vi "SQM160 Comm.vi"() -> (0 "TEMPSTRG":string="!#@O7")   [LabVIEW 2023]
panel:
  out "Shutter":bool
  out "COMPLETE MESSAGE 9":string
  out "CRC2 6":string
  out "CRC1 6":string
  out "Boolean array 6":bool[](array[boolean])
  in  "CRC 14":i16 format="%.0x"
  in  "TEMPCRC 6":i16=16383 format="%.0x"
  out "x-y*floor(x/y) 6":i32
  out "floor(x/y) 6":i32
  out "TEMPSTRG 9":string="!#@O7"
  out "COMPLETE MESSAGE 6":string
  out "CRC2 5":string
  out "CRC1 5":string
  out "Boolean array 5":bool[](array[boolean])
  in  "CRC 11":i16 format="%.0x"
  in  "TEMPCRC 5":i16=16383 format="%.0x"
  out "x-y*floor(x/y) 5":i32
  out "floor(x/y) 5":i32
  out "TEMPSTRG 7":string="!#@O7"
  out "CRC2 4":string
  out "CRC1 4":string
  out "Boolean array 4":bool[](array[boolean])
  in  "CRC 8":i16 format="%.0x"
  in  "TEMPCRC 4":i16=16383 format="%.0x"
  out "x-y*floor(x/y) 4":i32
  out "floor(x/y) 4":i32
  out "TEMPSTRG 5":string="!#@O7"
  out "error code 8":i32 format="%.0x"
  out "error code 7":i32
  out "COMPLETE MESSAGE 4":string
  out "COMPLETE MESSAGE 3":string
  out "CRC2 3":string
  out "CRC1 3":string
  out "Boolean array 3":bool[](array[boolean])
  in  "CRC 5":i16 format="%.0x"
  in  "TEMPCRC 3":i16=16383 format="%.0x"
  out "x-y*floor(x/y) 3":i32
  out "floor(x/y) 3":i32
  out "TEMPSTRG 3":string="!#@O7"
  out "error code 6":i32 format="%.0x"
  out "error code 5":i32
  out "COMPLETE MESSAGE 2":string
  out "CRC2 2":string
  out "CRC1 2":string
  out "TEMPSTRG 2":string="!#@O7"
  out "Boolean array 2":bool[](array[boolean])
  out "first subarray 2":bool[](array[boolean])
  out "second subarray 2":bool[](array[boolean])
  in  "CRC 2":i16 format="%.0x"
  in  "TEMPCRC 2":i16=16383 format="%.0x"
  out "x-y*floor(x/y) 2":i32
  out "floor(x/y) 2":i32
  in  "CH2 FREQUENCY CMD":string="P2"
  in  "CH1 FREQUENCY CMD":string="P1"
  in  "CH2 THICNESS CMD":string="N2"
  in  "CH1 THICKNESS CMD":string="N1"
  in  "CH2  RATE CMD":string="L2"
  out "STATUS":string
  out "error code 4":i32
  out "THICKNESS 2":string="N/A"
  out "FREQUENCY 2":string="N/A"
  out "RATE 2":string="N/A"
  out "FREQUENCY 1":string="N/A"
  out "THICNESS 1":string="N/A"
  out "RATE 1":string="N/A"
  in  "START/STOP":bool
  in  "BAUD RATE":u16(ring)=3 items=["2400", "4800", "9600", "19200", "38400"]
  out "Output Array":string[](array[string])
  out "error code 3":i32 format="%.0x"
  out "error code 2":i32
  out "error code":i32
  in  "COM PORT":u16(ring) items=["COM 1", "COM 2"]
  in  "INIT PORT":bool
  out "COMPLETE MESSAGE":string
  out "CRC2":string
  out "floor(x/y)":i32
  out "x-y*floor(x/y)":i32
  out "CRC1":string
  out "second subarray":bool[](array[boolean])
  out "first subarray":bool[](array[boolean])
  out "Boolean array":bool[](array[boolean])
  in  "CH1 RATE CMD":string="L1"
  in  "TEMPCRC":i16=16383 format="%.0x"
  in  "CRC":i16 format="%.0x"
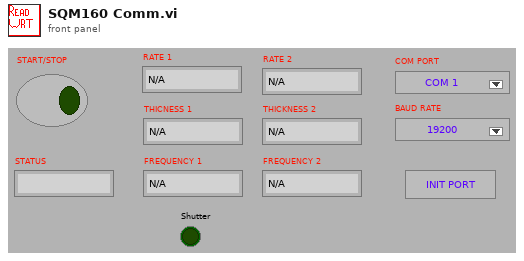
[diagram p1: front panel]
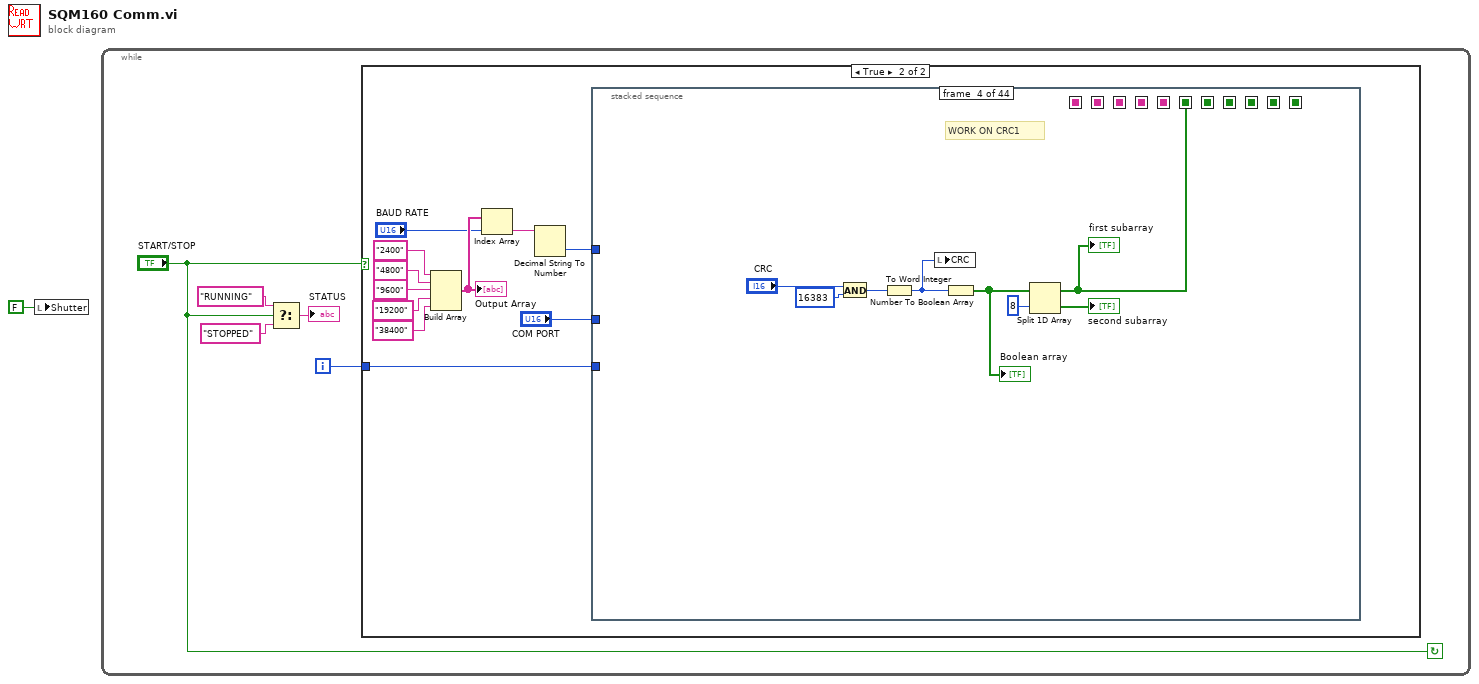
[diagram p0: block diagram]
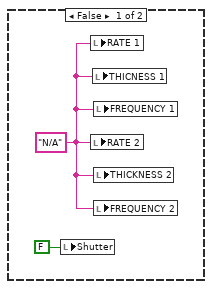
[diagram p2: hidden frame]
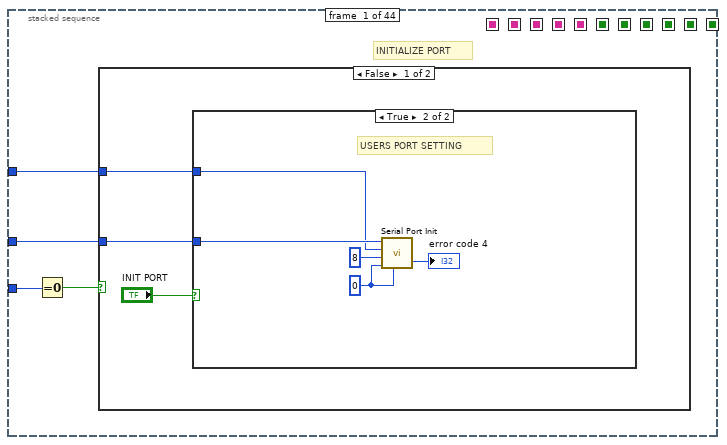
[diagram p3: hidden frame]
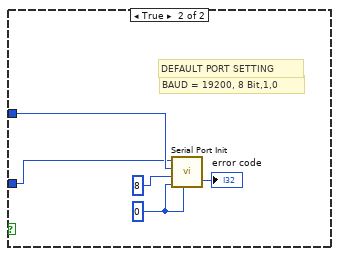
[diagram p5: hidden frame]
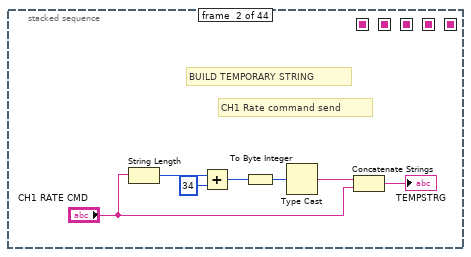
[diagram p6: hidden frame]
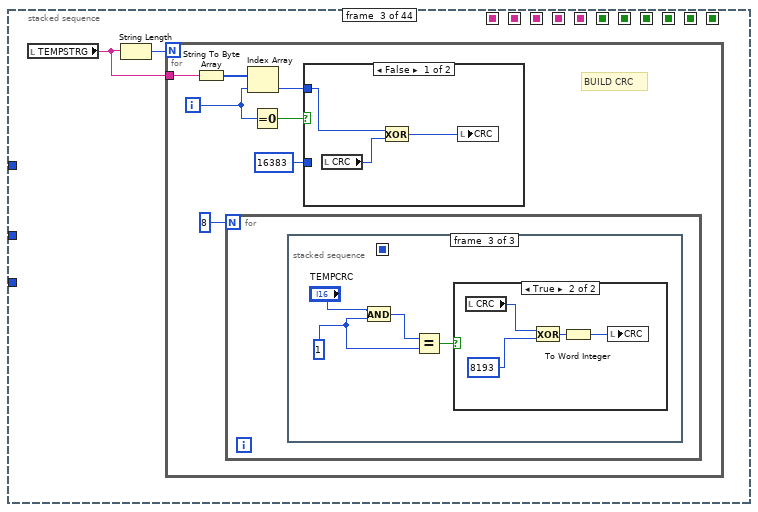
[diagram p7: hidden frame]
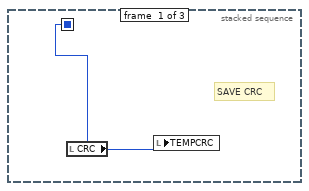
[diagram p8: hidden frame]
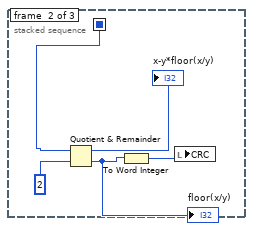
[diagram p9: hidden frame]
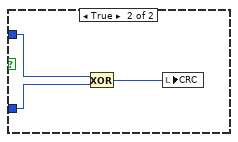
[diagram p11: hidden frame]
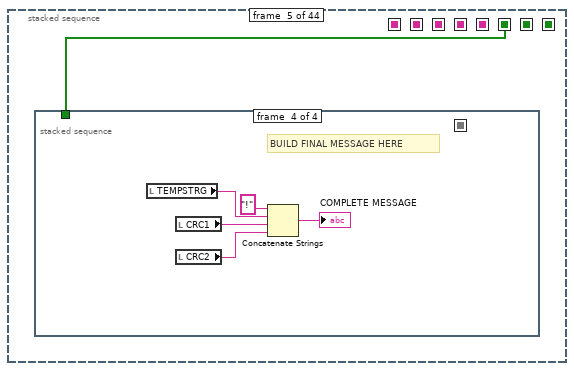
[diagram p12: hidden frame]
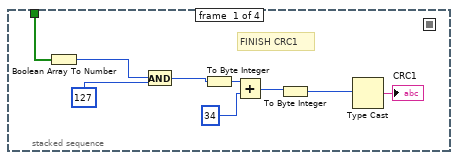
[diagram p13: hidden frame]
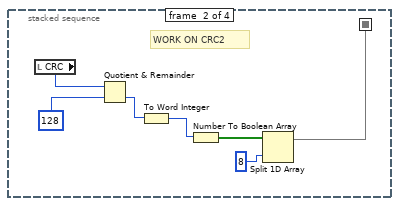
[diagram p14: hidden frame]
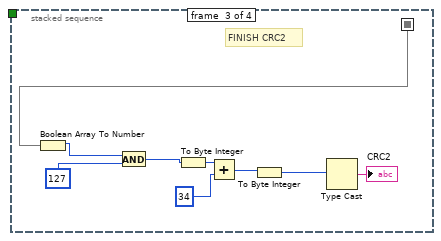
[diagram p15: hidden frame]
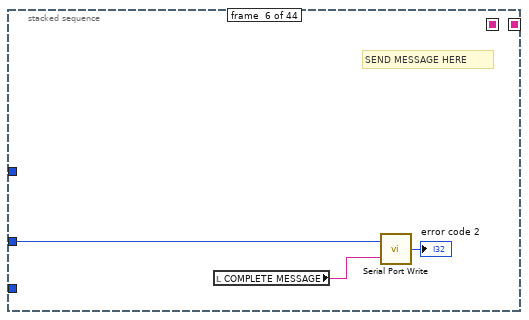
[diagram p16: hidden frame]
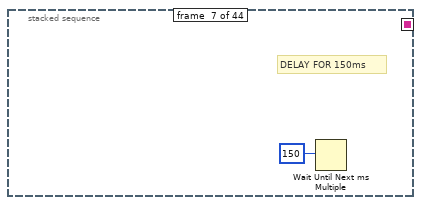
[diagram p17: hidden frame]
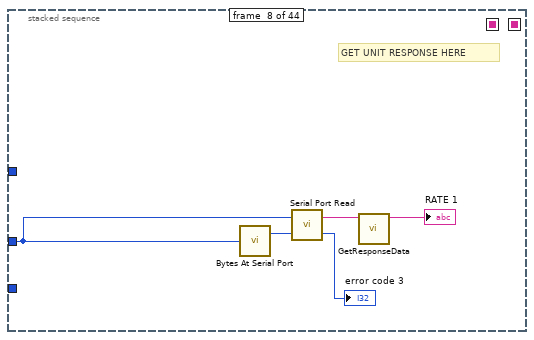
[diagram p18: hidden frame]
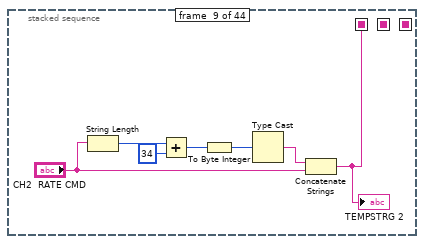
[diagram p19: hidden frame]
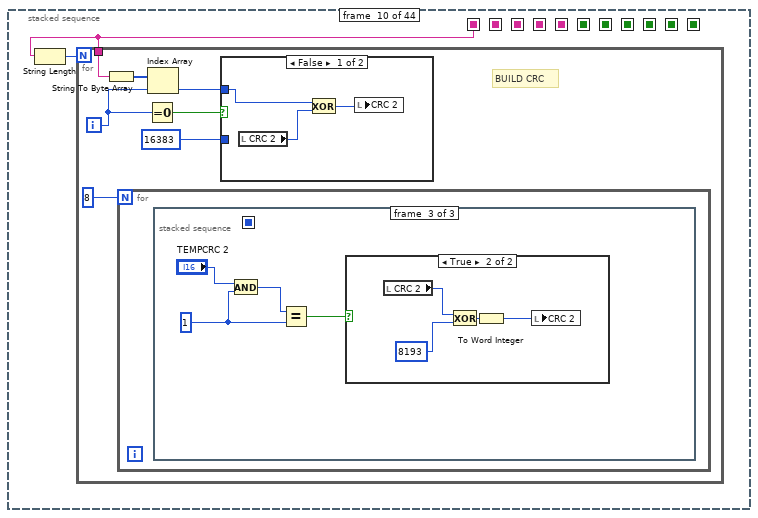
[diagram p20: hidden frame]
diagram:
  n1 = local write "Shutter"(FALSE ("Shutter")) -> ()
  n2 = while {
    i -> [w6]
    stop <- "START/STOP" continue-if-true
    n3 = Select(t="RUNNING", s="START/STOP", f="STOPPED") -> (s? t:f=→"STATUS":string)
    n4 = case shown="True" "START/STOP" {
      tunnel: w6 -> [_ w18]
      frame False {
        w8 = "N/A"
        n5 = local write "Shutter"(FALSE ("Shutter")) -> ()
        n6 = local write "RATE 1"(w8) -> ()
        n7 = local write "RATE 2"(w8) -> ()
        n8 = local write "THICNESS 1"(w8) -> ()
        n9 = local write "FREQUENCY 1"(w8) -> ()
        n10 = local write "THICKNESS 2"(w8) -> ()
        n11 = local write "FREQUENCY 2"(w8) -> ()
      }
      frame True {
        n12 = Build Array("2400", "4800", "9600", "19200", "38400") -> (w12:string[])
        "Output Array" <- w12
        n13 = Index Array(array=w12, index="BAUD RATE") -> (element=w11:string)
        n14 = Decimal String To Number(string=w11) -> (number=w9:i32)  [unwired: 2 in, 1 out]
        n15 = stacked-sequence {
          seq-local: [_ _ _ w77 _ _ _ _ _ _ _ _ _ _ _ _ _ _ _ _ _ _ _ _ _ _ _ _ _ _ _ _ _ _ _ _ _ _ _ _ _ _ _ _] -> [_ _ _ _ w81 _ _ _ _ _ _ _ _ _ _ _ _ _ _ _ _ _ _ _ _ _ _ _ _ _ _ _ _ _ _ _ _ _ _ _ _ _ _ _]
          seq-local: [_ _ _ _ _ _ _ _ w121 _ _ _ _ _ _ _ _ _ _ _ _ _ _ _ _ _ _ _ _ _ _ _ _ _ _ _ _ _ _ _ _ _ _ _] -> [_ _ _ _ _ _ _ _ _ w128 _ _ _ _ _ _ _ _ _ _ _ _ _ _ _ _ _ _ _ _ _ _ _ _ _ _ _ _ _ _ _ _ _ _]
          seq-local: [_ _ _ _ _ _ _ _ _ _ w159 _ _ _ _ _ _ _ _ _ _ _ _ _ _ _ _ _ _ _ _ _ _ _ _ _ _ _ _ _ _ _ _ _] -> [_ _ _ _ _ _ _ _ _ _ _ w165 _ _ _ _ _ _ _ _ _ _ _ _ _ _ _ _ _ _ _ _ _ _ _ _ _ _ _ _ _ _ _ _]
          seq-local: [_ _ _ _ _ _ _ _ _ _ _ _ _ _ _ w206 _ _ _ _ _ _ _ _ _ _ _ _ _ _ _ _ _ _ _ _ _ _ _ _ _ _ _ _] -> [_ _ _ _ _ _ _ _ _ _ _ _ _ _ _ _ w212 _ _ _ _ _ _ _ _ _ _ _ _ _ _ _ _ _ _ _ _ _ _ _ _ _ _ _]
          seq-local: [_ _ _ _ _ _ _ _ _ _ _ _ _ _ _ _ _ w242 _ _ _ _ _ _ _ _ _ _ _ _ _ _ _ _ _ _ _ _ _ _ _ _ _ _] -> [_ _ _ _ _ _ _ _ _ _ _ _ _ _ _ _ _ _ w248 _ _ _ _ _ _ _ _ _ _ _ _ _ _ _ _ _ _ _ _ _ _ _ _ _]
          seq-local: [_ _ _ _ _ _ _ _ _ _ _ _ _ _ _ _ _ _ _ _ _ _ w288 _ _ _ _ _ _ _ _ _ _ _ _ _ _ _ _ _ _ _ _ _] -> [_ _ _ _ _ _ _ _ _ _ _ _ _ _ _ _ _ _ _ _ _ _ _ w295 _ _ _ _ _ _ _ _ _ _ _ _ _ _ _ _ _ _ _ _]
          seq-local: [_ _ _ _ _ _ _ _ _ _ _ _ _ _ _ _ _ _ _ _ _ _ _ _ w325 _ _ _ _ _ _ _ _ _ _ _ _ _ _ _ _ _ _ _] -> [_ _ _ _ _ _ _ _ _ _ _ _ _ _ _ _ _ _ _ _ _ _ _ _ _ w331 _ _ _ _ _ _ _ _ _ _ _ _ _ _ _ _ _ _]
          seq-local: [_ _ _ _ _ _ _ _ _ _ _ _ _ _ _ _ _ _ _ _ _ _ _ _ _ _ _ _ _ w369 _ _ _ _ _ _ _ _ _ _ _ _ _ _] -> [_ _ _ _ _ _ _ _ _ _ _ _ _ _ _ _ _ _ _ _ _ _ _ _ _ _ _ _ _ _ w376 _ _ _ _ _ _ _ _ _ _ _ _ _]
          seq-local: [_ _ _ _ _ _ _ _ _ _ _ _ _ _ _ _ _ _ _ _ _ _ _ _ _ _ _ _ _ _ _ w406 _ _ _ _ _ _ _ _ _ _ _ _] -> [_ _ _ _ _ _ _ _ _ _ _ _ _ _ _ _ _ _ _ _ _ _ _ _ _ _ _ _ _ _ _ _ w412 _ _ _ _ _ _ _ _ _ _ _]
          seq-local: [_ _ _ _ _ _ _ _ _ _ _ _ _ _ _ _ _ _ _ _ _ _ _ _ _ _ _ _ _ _ _ _ _ _ _ _ w450 _ _ _ _ _ _ _] -> [_ _ _ _ _ _ _ _ _ _ _ _ _ _ _ _ _ _ _ _ _ _ _ _ _ _ _ _ _ _ _ _ _ _ _ _ _ w457 _ _ _ _ _ _]
          seq-local: [_ _ _ _ _ _ _ _ _ _ _ _ _ _ _ _ _ _ _ _ _ _ _ _ _ _ _ _ _ _ _ _ _ _ _ _ _ _ w488 _ _ _ _ _] -> [_ _ _ _ _ _ _ _ _ _ _ _ _ _ _ _ _ _ _ _ _ _ _ _ _ _ _ _ _ _ _ _ _ _ _ _ _ _ _ w493 _ _ _ _]
          tunnel: "COM PORT" -> [w23 _ _ _ _ w112 _ w118 _ _ _ _ w196 _ w202 _ _ _ _ w279 _ w285 _ _ _ _ w362 _ w368 _ _ _ _ w443 _ w448 _ _ _ _ w524 _ w529 w531]
          tunnel: w18 -> [w22 _ _ _ _ _ _ _ _ _ _ _ _ _ _ _ _ _ _ _ _ _ _ _ _ _ _ _ _ _ _ _ _ _ _ _ _ _ _ _ _ _ _ _]
          tunnel: w9 -> [w20 _ _ _ _ _ _ _ _ _ _ _ _ _ _ _ _ _ _ _ _ _ _ _ _ _ _ _ _ _ _ _ _ _ _ _ _ _ _ _ _ _ _ _]
          frame #0 {
            # "INITIALIZE PORT"
            n16 = Equal To 0?(x=w22) -> (x = 0?=w21:bool)
            n17 = case shown="False" w21 {
              tunnel: w20 -> [w24 w36]
              tunnel: w23 -> [w25 w34]
              frame False {
                n18 = case shown="True" "INIT PORT" {
                  tunnel: w25 -> [_ w28]
                  tunnel: w24 -> [_ w27]
                  frame False {
                  }
                  frame True {
                    w30 = 0
                    # "USERS PORT SETTING"
                    n19 = call <vilib>:"Serial Port Init.vi"("parity"=w30, "stop bits"=w30, "data bits"=8, "baud rate"=w27, "port number"=w28) -> ("error code"=→"error code 4":i32)  [unwired: 2 in]
                  }
                }
              }
              frame True {
                w33 = 0
                # "BAUD = 19200, 8 Bit,1,0"
                # "DEFAULT PORT SETTING"
                n20 = call <vilib>:"Serial Port Init.vi"("parity"=w33, "stop bits"=w33, "data bits"=8, "baud rate"=w36, "port number"=w34) -> ("error code"=→"error code":i32)  [unwired: 2 in]
              }
            }
          }
          frame #1 {
            # "CH1 Rate command send"
            # "BUILD TEMPORARY STRING"
            n21 = String Length(string="CH1 RATE CMD") -> (length=w43:i32)
            n22 = Add(x=w43, y=34) -> (x+y=w39:i32)
            n23 = To Byte Integer(number=w39) -> (8bit integer=w40:i8)
            n24 = Type Cast(x=w40) -> (*(type *) &x=w38:string)  [unwired: 1 in]
            n25 = Concatenate Strings(w38, "CH1 RATE CMD") -> (→"TEMPSTRG":string)
          }
          frame #2 {
            n26 = local read "TEMPSTRG"() -> (w45:string)
            n27 = String Length(string=w45) -> (length=w44:i32)
            n28 = for {
              N: w44 -> [_]
              tunnel: w45 -> [w49]
              i -> [w52]
              # "BUILD CRC"
              n29 = String To Byte Array(string=w49) -> (unsigned byte array=w48:u8[])
              n30 = for {
                N: 8 -> [_]
                n31 = stacked-sequence {
                  seq-local: [w53 _ _] -> [_ w58 _]
                  frame #0 {
                    # "SAVE CRC"
                    n32 = local read "CRC"() -> (w53:i16)
                    n33 = local write "TEMPCRC"(w53) -> ()
                  }
                  frame #1 {
                    n34 = Quotient & Remainder(x=w58, y=2) -> (x-y*floor(x/y)=→"x-y*floor(x/y)":i32, floor(x/y)=w54:i32)
                    "floor(x/y)" <- w54
                    n35 = To Word Integer(number=w54) -> (16bit integer=w56:i16)
                    n36 = local write "CRC"(w56) -> ()
                  }
                  frame #2 {
                    w60 = 1
                    n37 = And(x="TEMPCRC", y=w60) -> (x .and. y?=w61:i32)
                    n38 = Equal?(x=w61, y=w60) -> (x = y?=w59:bool)
                    n39 = case shown="True" w59 {
                      frame False {
                      }
                      frame True {
                        n40 = local read "CRC"() -> (w64:i16)
                        n41 = Exclusive Or(1:8193, 2:w64) -> (0:w63:i32)
                        n42 = To Word Integer(number=w63) -> (16bit integer=w66:i16)
                        n43 = local write "CRC"(w66) -> ()
                      }
                    }
                  }
                }
              }
              n44 = Index Array(array=w48, index=w52) -> (element=w46:u8)
              n45 = Equal To 0?(x=w52) -> (x = 0?=w51:bool)
              n46 = case shown="False" w51 {
                tunnel: 16383 -> [_ w72]
                tunnel: w46 -> [w69 w71]
                frame False {
                  n47 = local read "CRC"() -> (w68:i16)
                  n48 = Exclusive Or(1:w68, 2:w69) -> (0:w67:i16)
                  n49 = local write "CRC"(w67) -> ()
                }
                frame True {
                  n50 = Exclusive Or(1:w72, 2:w71) -> (0:w70:i32)
                  n51 = local write "CRC"(w70) -> ()
                }
              }
            }
          }
          frame #3 {
            # "WORK ON CRC1"
            n52 = And(x="CRC", y=16383) -> (x .and. y?=w74:i32)
            n53 = To Word Integer(number=w74) -> (16bit integer=w73:i16)
            n54 = local write "CRC"(w73) -> ()
            n55 = Number To Boolean Array(number=w73) -> (Boolean array=w80:bool[])
            "Boolean array" <- w80
            n56 = Split 1D Array(array=w80, index=8) -> (first subarray=w77:bool[], second subarray=→"second subarray":bool[])
            "first subarray" <- w77
          }
          frame #4 {
            n57 = stacked-sequence {
              seq-local: [_ w91 _ _] -> [_ _ w98 _]
              tunnel: w81 -> [w82 _ _ _]
              frame #0 {
                # "FINISH CRC1"
                n58 = Boolean Array To Number(Boolean array=w82) -> (number=w83:u32)
                n59 = And(x=w83, y=127) -> (x .and. y?=w84:u32)
                n60 = To Byte Integer(number=w84) -> (8bit integer=w86:i8)
                n61 = Add(x=w86, y=34) -> (x+y=w88:i32)
                n62 = To Byte Integer(number=w88) -> (8bit integer=w87:i8)
                n63 = Type Cast(x=w87) -> (*(type *) &x=→"CRC1":string)  [unwired: 1 in]
              }
              frame #1 {
                # "WORK ON CRC2"
                n64 = local read "CRC"() -> (w97:i16)
                n65 = Quotient & Remainder(x=w97, y=128) -> (floor(x/y)=w94:i32)  [unwired: 1 out]
                n66 = To Word Integer(number=w94) -> (16bit integer=w93:i16)
                n67 = Number To Boolean Array(number=w93) -> (Boolean array=w92:bool[])
                n68 = Split 1D Array(array=w92, index=8) -> (first subarray=w91:bool[])  [unwired: 1 out]
              }
              frame #2 {
                # "FINISH CRC2"
                n69 = Boolean Array To Number(Boolean array=w98) -> (number=w99:u32)
                n70 = And(x=w99, y=127) -> (x .and. y?=w106:u32)
                n71 = To Byte Integer(number=w106) -> (8bit integer=w104:i8)
                n72 = Add(x=w104, y=34) -> (x+y=w102:i32)
                n73 = To Byte Integer(number=w102) -> (8bit integer=w103:i8)
                n74 = Type Cast(x=w103) -> (*(type *) &x=→"CRC2":string)  [unwired: 1 in]
              }
              frame #3 {
                # "BUILD FINAL MESSAGE HERE"
                n75 = local read "TEMPSTRG"() -> (w110:string)
                n76 = local read "CRC1"() -> (w109:string)
                n77 = local read "CRC2"() -> (w108:string)
                n78 = Concatenate Strings("!", w110, w109, w108) -> (→"COMPLETE MESSAGE":string)
              }
            }
          }
          frame #5 {
            # "SEND MESSAGE HERE"
            n79 = local read "COMPLETE MESSAGE"() -> (w114:string)
            n80 = call <vilib>:"Serial Port Write.vi"("string to write"=w114, "port number"=w112) -> ("error code"=→"error code 2":i32)
          }
          frame #6 {
            # "DELAY FOR 150ms"
            n81 = Wait Until Next ms Multiple(millisecond multiple=150) -> ()  [unwired: 1 out]
          }
          frame #7 {
            # "GET UNIT RESPONSE HERE"
            n82 = call <vilib>:"Bytes At Serial Port.vi"("port number"=w118) -> ("byte count"=w119:u32)  [unwired: 1 out]
            n83 = call <vilib>:"Serial Port Read.vi"("requested byte count"=w119, "port number"=w118) -> ("error code"=→"error code 3":i32, "string read"=w117:string)
            n84 = call "GetResponseData.vi"("string read"=w117) -> ("replaced substring"=→"RATE 1":string)  [unwired: 10 in]
          }
          frame #8 {
            n85 = String Length(string="CH2  RATE CMD") -> (length=w127:i32)
            n86 = Add(x=w127, y=34) -> (x+y=w124:i32)
            n87 = To Byte Integer(number=w124) -> (8bit integer=w125:i8)
            n88 = Type Cast(x=w125) -> (*(type *) &x=w122:string)  [unwired: 1 in]
            n89 = Concatenate Strings(w122, "CH2  RATE CMD") -> (w121:string)
            "TEMPSTRG 2" <- w121
          }
          frame #9 {
            n90 = String Length(string=w128) -> (length=w129:i32)
            n91 = for {
              N: w129 -> [_]
              tunnel: w128 -> [w133]
              i -> [w136]
              # "BUILD CRC"
              n92 = String To Byte Array(string=w133) -> (unsigned byte array=w132:u8[])
              n93 = for {
                N: 8 -> [_]
                n94 = stacked-sequence {
                  seq-local: [w137 _ _] -> [_ w142 _]
                  frame #0 {
                    # "SAVE CRC"
                    n95 = local read "CRC 2"() -> (w137:i16)
                    n96 = local write "TEMPCRC 2"(w137) -> ()
                  }
                  frame #1 {
                    n97 = Quotient & Remainder(x=w142, y=2) -> (x-y*floor(x/y)=→"x-y*floor(x/y) 2":i32, floor(x/y)=w138:i32)
                    "floor(x/y) 2" <- w138
                    n98 = To Word Integer(number=w138) -> (16bit integer=w140:i16)
                    n99 = local write "CRC 2"(w140) -> ()
                  }
                  frame #2 {
                    w144 = 1
                    n100 = And(x="TEMPCRC 2", y=w144) -> (x .and. y?=w145:i32)
                    n101 = Equal?(x=w145, y=w144) -> (x = y?=w143:bool)
                    n102 = case shown="True" w143 {
                      frame False {
                      }
                      frame True {
                        n103 = local read "CRC 2"() -> (w148:i16)
                        n104 = Exclusive Or(1:8193, 2:w148) -> (0:w147:i32)
                        n105 = To Word Integer(number=w147) -> (16bit integer=w150:i16)
                        n106 = local write "CRC 2"(w150) -> ()
                      }
                    }
                  }
                }
              }
              n107 = Equal To 0?(x=w136) -> (x = 0?=w135:bool)
              n108 = Index Array(array=w132, index=w136) -> (element=w130:u8)
              n109 = case shown="False" w135 {
                tunnel: 16383 -> [_ w156]
                tunnel: w130 -> [w153 w155]
                frame False {
                  n110 = local read "CRC 2"() -> (w152:i16)
                  n111 = Exclusive Or(1:w152, 2:w153) -> (0:w151:i16)
                  n112 = local write "CRC 2"(w151) -> ()
                }
                frame True {
                  n113 = Exclusive Or(1:w156, 2:w155) -> (0:w154:i32)
                  n114 = local write "CRC 2"(w154) -> ()
                }
              }
            }
          }
          frame #10 {
            n115 = And(x="CRC 2", y=16383) -> (x .and. y?=w160:i32)
            n116 = To Word Integer(number=w160) -> (16bit integer=w157:i16)
            n117 = local write "CRC 2"(w157) -> ()
            n118 = Number To Boolean Array(number=w157) -> (Boolean array=w164:bool[])
            "Boolean array 2" <- w164
            n119 = Split 1D Array(array=w164, index=8) -> (first subarray=w159:bool[], second subarray=→"second subarray 2":bool[])
            "first subarray 2" <- w159
          }
          frame #11 {
            n120 = stacked-sequence {
              seq-local: [_ w175 _ _] -> [_ _ w182 _]
              tunnel: w165 -> [w166 _ _ _]
              frame #0 {
                # "FINISH CRC1"
                n121 = Boolean Array To Number(Boolean array=w166) -> (number=w167:u32)
                n122 = And(x=w167, y=127) -> (x .and. y?=w168:u32)
                n123 = To Byte Integer(number=w168) -> (8bit integer=w170:i8)
                n124 = Add(x=w170, y=34) -> (x+y=w172:i32)
                n125 = To Byte Integer(number=w172) -> (8bit integer=w171:i8)
                n126 = Type Cast(x=w171) -> (*(type *) &x=→"CRC1 2":string)  [unwired: 1 in]
              }
              frame #1 {
                # "WORK ON CRC2"
                n127 = local read "CRC 2"() -> (w181:i16)
                n128 = Quotient & Remainder(x=w181, y=128) -> (floor(x/y)=w178:i32)  [unwired: 1 out]
                n129 = To Word Integer(number=w178) -> (16bit integer=w177:i16)
                n130 = Number To Boolean Array(number=w177) -> (Boolean array=w176:bool[])
                n131 = Split 1D Array(array=w176, index=8) -> (first subarray=w175:bool[])  [unwired: 1 out]
              }
              frame #2 {
                # "FINISH CRC2"
                n132 = Boolean Array To Number(Boolean array=w182) -> (number=w183:u32)
                n133 = And(x=w183, y=127) -> (x .and. y?=w190:u32)
                n134 = To Byte Integer(number=w190) -> (8bit integer=w188:i8)
                n135 = Add(x=w188, y=34) -> (x+y=w186:i32)
                n136 = To Byte Integer(number=w186) -> (8bit integer=w187:i8)
                n137 = Type Cast(x=w187) -> (*(type *) &x=→"CRC2 2":string)  [unwired: 1 in]
              }
              frame #3 {
                # "BUILD FINAL MESSAGE HERE"
                n138 = local read "TEMPSTRG 2"() -> (w194:string)
                n139 = local read "CRC1 2"() -> (w193:string)
                n140 = local read "CRC2 2"() -> (w192:string)
                n141 = Concatenate Strings("!", w194, w193, w192) -> (→"COMPLETE MESSAGE 2":string)
              }
            }
          }
          frame #12 {
            n142 = local read "COMPLETE MESSAGE 2"() -> (w197:string)
            n143 = call <vilib>:"Serial Port Write.vi"("string to write"=w197, "port number"=w196) -> ("error code"=→"error code 5":i32)
          }
          frame #13 {
            # "DELAY FOR 150ms"
            n144 = Wait Until Next ms Multiple(millisecond multiple=150) -> ()  [unwired: 1 out]
          }
          frame #14 {
            n145 = call <vilib>:"Bytes At Serial Port.vi"("port number"=w202) -> ("byte count"=w203:u32)  [unwired: 1 out]
            n146 = call <vilib>:"Serial Port Read.vi"("requested byte count"=w203, "port number"=w202) -> ("error code"=→"error code 6":i32, "string read"=w201:string)
            n147 = call "GetResponseData.vi"("string read"=w201) -> ("replaced substring"=→"RATE 2":string)  [unwired: 10 in]
          }
          frame #15 {
            n148 = String Length(string="CH1 THICKNESS CMD") -> (length=w211:i32)
            n149 = Add(x=w211, y=34) -> (x+y=w208:i32)
            n150 = To Byte Integer(number=w208) -> (8bit integer=w209:i8)
            n151 = Type Cast(x=w209) -> (*(type *) &x=w207:string)  [unwired: 1 in]
            n152 = Concatenate Strings(w207, "CH1 THICKNESS CMD") -> (w206:string)
            "TEMPSTRG 3" <- w206
          }
          frame #16 {
            n153 = String Length(string=w212) -> (length=w213:i32)
            n154 = for {
              N: w213 -> [_]
              tunnel: w212 -> [w217]
              i -> [w220]
              # "BUILD CRC"
              n155 = String To Byte Array(string=w217) -> (unsigned byte array=w216:u8[])
              n156 = for {
                N: 8 -> [_]
                n157 = stacked-sequence {
                  seq-local: [w221 _ _] -> [_ w226 _]
                  frame #0 {
                    # "SAVE CRC"
                    n158 = local read "CRC 5"() -> (w221:i16)
                    n159 = local write "TEMPCRC 3"(w221) -> ()
                  }
                  frame #1 {
                    n160 = Quotient & Remainder(x=w226, y=2) -> (x-y*floor(x/y)=→"x-y*floor(x/y) 3":i32, floor(x/y)=w222:i32)
                    "floor(x/y) 3" <- w222
                    n161 = To Word Integer(number=w222) -> (16bit integer=w224:i16)
                    n162 = local write "CRC 5"(w224) -> ()
                  }
                  frame #2 {
                    w228 = 1
                    n163 = And(x="TEMPCRC 3", y=w228) -> (x .and. y?=w229:i32)
                    n164 = Equal?(x=w229, y=w228) -> (x = y?=w227:bool)
                    n165 = case shown="True" w227 {
                      frame False {
                      }
                      frame True {
                        n166 = local read "CRC 5"() -> (w232:i16)
                        n167 = Exclusive Or(1:8193, 2:w232) -> (0:w231:i32)
                        n168 = To Word Integer(number=w231) -> (16bit integer=w234:i16)
                        n169 = local write "CRC 5"(w234) -> ()
                      }
                    }
                  }
                }
              }
              n170 = Index Array(array=w216, index=w220) -> (element=w214:u8)
              n171 = Equal To 0?(x=w220) -> (x = 0?=w219:bool)
              n172 = case shown="False" w219 {
                tunnel: 16383 -> [_ w240]
                tunnel: w214 -> [w237 w239]
                frame False {
                  n173 = local read "CRC 5"() -> (w236:i16)
                  n174 = Exclusive Or(1:w236, 2:w237) -> (0:w235:i16)
                  n175 = local write "CRC 5"(w235) -> ()
                }
                frame True {
                  n176 = Exclusive Or(1:w240, 2:w239) -> (0:w238:i32)
                  n177 = local write "CRC 5"(w238) -> ()
                }
              }
            }
          }
          frame #17 {
            n178 = And(x="CRC 5", y=16383) -> (x .and. y?=w244:i32)
            n179 = To Word Integer(number=w244) -> (16bit integer=w243:i16)
            n180 = local write "CRC 5"(w243) -> ()
            n181 = Number To Boolean Array(number=w243) -> (Boolean array=w247:bool[])
            "Boolean array 3" <- w247
            n182 = Split 1D Array(array=w247, index=8) -> (first subarray=w242:bool[])  [unwired: 1 out]
          }
          frame #18 {
            n183 = stacked-sequence {
              seq-local: [_ w258 _ _] -> [_ _ w265 _]
              tunnel: w248 -> [w249 _ _ _]
              frame #0 {
                # "FINISH CRC1"
                n184 = Boolean Array To Number(Boolean array=w249) -> (number=w250:u32)
                n185 = And(x=w250, y=127) -> (x .and. y?=w251:u32)
                n186 = To Byte Integer(number=w251) -> (8bit integer=w253:i8)
                n187 = Add(x=w253, y=34) -> (x+y=w255:i32)
                n188 = To Byte Integer(number=w255) -> (8bit integer=w254:i8)
                n189 = Type Cast(x=w254) -> (*(type *) &x=→"CRC1 3":string)  [unwired: 1 in]
              }
              frame #1 {
                # "WORK ON CRC2"
                n190 = local read "CRC 5"() -> (w264:i16)
                n191 = Quotient & Remainder(x=w264, y=128) -> (floor(x/y)=w261:i32)  [unwired: 1 out]
                n192 = To Word Integer(number=w261) -> (16bit integer=w260:i16)
                n193 = Number To Boolean Array(number=w260) -> (Boolean array=w259:bool[])
                n194 = Split 1D Array(array=w259, index=8) -> (first subarray=w258:bool[])  [unwired: 1 out]
              }
              frame #2 {
                # "FINISH CRC2"
                n195 = Boolean Array To Number(Boolean array=w265) -> (number=w266:u32)
                n196 = And(x=w266, y=127) -> (x .and. y?=w273:u32)
                n197 = To Byte Integer(number=w273) -> (8bit integer=w271:i8)
                n198 = Add(x=w271, y=34) -> (x+y=w269:i32)
                n199 = To Byte Integer(number=w269) -> (8bit integer=w270:i8)
                n200 = Type Cast(x=w270) -> (*(type *) &x=→"CRC2 3":string)  [unwired: 1 in]
              }
              frame #3 {
                # "BUILD FINAL MESSAGE HERE"
                n201 = local read "TEMPSTRG 3"() -> (w277:string)
                n202 = local read "CRC1 3"() -> (w276:string)
                n203 = local read "CRC2 3"() -> (w275:string)
                n204 = Concatenate Strings("!", w277, w276, w275) -> (→"COMPLETE MESSAGE 3":string)
              }
            }
          }
          frame #19 {
            n205 = local read "COMPLETE MESSAGE 3"() -> (w280:string)
            n206 = call <vilib>:"Serial Port Write.vi"("string to write"=w280, "port number"=w279) -> ("error code"=→"error code 7":i32)
          }
          frame #20 {
            # "DELAY FOR 150ms"
            n207 = Wait Until Next ms Multiple(millisecond multiple=150) -> ()  [unwired: 1 out]
          }
          frame #21 {
            n208 = call <vilib>:"Bytes At Serial Port.vi"("port number"=w285) -> ("byte count"=w286:u32)  [unwired: 1 out]
            n209 = call <vilib>:"Serial Port Read.vi"("requested byte count"=w286, "port number"=w285) -> ("error code"=→"error code 8":i32, "string read"=w284:string)
            n210 = call "GetResponseData.vi"("string read"=w284) -> ("replaced substring"=→"THICNESS 1":string)  [unwired: 10 in]
          }
          frame #22 {
            n211 = String Length(string="CH2 THICNESS CMD") -> (length=w294:i32)
            n212 = Add(x=w294, y=34) -> (x+y=w291:i32)
            n213 = To Byte Integer(number=w291) -> (8bit integer=w292:i8)
            n214 = Type Cast(x=w292) -> (*(type *) &x=w290:string)  [unwired: 1 in]
            n215 = Concatenate Strings(w290, "CH2 THICNESS CMD") -> (w288:string)
            "TEMPSTRG 5" <- w288
          }
          frame #23 {
            n216 = String Length(string=w295) -> (length=w296:i32)
            n217 = for {
              N: w296 -> [_]
              tunnel: w295 -> [w300]
              i -> [w303]
              # "BUILD CRC"
              n218 = String To Byte Array(string=w300) -> (unsigned byte array=w299:u8[])
              n219 = Equal To 0?(x=w303) -> (x = 0?=w302:bool)
              n220 = Index Array(array=w299, index=w303) -> (element=w297:u8)
              n221 = for {
                N: 8 -> [_]
                n222 = stacked-sequence {
                  seq-local: [w304 _ _] -> [_ w309 _]
                  frame #0 {
                    # "SAVE CRC"
                    n223 = local read "CRC 8"() -> (w304:i16)
                    n224 = local write "TEMPCRC 4"(w304) -> ()
                  }
                  frame #1 {
                    n225 = Quotient & Remainder(x=w309, y=2) -> (x-y*floor(x/y)=→"x-y*floor(x/y) 4":i32, floor(x/y)=w305:i32)
                    "floor(x/y) 4" <- w305
                    n226 = To Word Integer(number=w305) -> (16bit integer=w307:i16)
                    n227 = local write "CRC 8"(w307) -> ()
                  }
                  frame #2 {
                    w311 = 1
                    n228 = And(x="TEMPCRC 4", y=w311) -> (x .and. y?=w312:i32)
                    n229 = Equal?(x=w312, y=w311) -> (x = y?=w310:bool)
                    n230 = case shown="True" w310 {
                      frame False {
                      }
                      frame True {
                        n231 = local read "CRC 8"() -> (w315:i16)
                        n232 = Exclusive Or(1:8193, 2:w315) -> (0:w314:i32)
                        n233 = To Word Integer(number=w314) -> (16bit integer=w317:i16)
                        n234 = local write "CRC 8"(w317) -> ()
                      }
                    }
                  }
                }
              }
              n235 = case shown="False" w302 {
                tunnel: 16383 -> [_ w323]
                tunnel: w297 -> [w320 w322]
                frame False {
                  n236 = local read "CRC 8"() -> (w319:i16)
                  n237 = Exclusive Or(1:w319, 2:w320) -> (0:w318:i16)
                  n238 = local write "CRC 8"(w318) -> ()
                }
                frame True {
                  n239 = Exclusive Or(1:w323, 2:w322) -> (0:w321:i32)
                  n240 = local write "CRC 8"(w321) -> ()
                }
              }
            }
          }
          frame #24 {
            n241 = And(x="CRC 8", y=16383) -> (x .and. y?=w327:i32)
            n242 = To Word Integer(number=w327) -> (16bit integer=w326:i16)
            n243 = local write "CRC 8"(w326) -> ()
            n244 = Number To Boolean Array(number=w326) -> (Boolean array=w330:bool[])
            "Boolean array 4" <- w330
            n245 = Split 1D Array(array=w330, index=8) -> (first subarray=w325:bool[])  [unwired: 1 out]
          }
          frame #25 {
            n246 = stacked-sequence {
              seq-local: [_ w341 _ _] -> [_ _ w348 _]
              tunnel: w331 -> [w332 _ _ _]
              frame #0 {
                # "FINISH CRC1"
                n247 = Boolean Array To Number(Boolean array=w332) -> (number=w333:u32)
                n248 = And(x=w333, y=127) -> (x .and. y?=w334:u32)
                n249 = To Byte Integer(number=w334) -> (8bit integer=w336:i8)
                n250 = Add(x=w336, y=34) -> (x+y=w338:i32)
                n251 = To Byte Integer(number=w338) -> (8bit integer=w337:i8)
                n252 = Type Cast(x=w337) -> (*(type *) &x=→"CRC1 4":string)  [unwired: 1 in]
              }
              frame #1 {
                # "WORK ON CRC2"
                n253 = local read "CRC 8"() -> (w347:i16)
                n254 = Quotient & Remainder(x=w347, y=128) -> (floor(x/y)=w344:i32)  [unwired: 1 out]
                n255 = To Word Integer(number=w344) -> (16bit integer=w343:i16)
                n256 = Number To Boolean Array(number=w343) -> (Boolean array=w342:bool[])
                n257 = Split 1D Array(array=w342, index=8) -> (first subarray=w341:bool[])  [unwired: 1 out]
              }
              frame #2 {
                # "FINISH CRC2"
                n258 = Boolean Array To Number(Boolean array=w348) -> (number=w349:u32)
                n259 = And(x=w349, y=127) -> (x .and. y?=w356:u32)
                n260 = To Byte Integer(number=w356) -> (8bit integer=w354:i8)
                n261 = Add(x=w354, y=34) -> (x+y=w352:i32)
                n262 = To Byte Integer(number=w352) -> (8bit integer=w353:i8)
                n263 = Type Cast(x=w353) -> (*(type *) &x=→"CRC2 4":string)  [unwired: 1 in]
              }
              frame #3 {
                # "BUILD FINAL MESSAGE HERE"
                n264 = local read "TEMPSTRG 5"() -> (w360:string)
                n265 = local read "CRC1 4"() -> (w359:string)
                n266 = local read "CRC2 4"() -> (w358:string)
                n267 = Concatenate Strings("!", w360, w359, w358) -> (→"COMPLETE MESSAGE 4":string)
              }
            }
          }
          frame #26 {
            n268 = local read "COMPLETE MESSAGE 4"() -> (w363:string)
            n269 = call <vilib>:"Serial Port Write.vi"("string to write"=w363, "port number"=w362) -> ()  [unwired: 1 out]
          }
          frame #27 {
            # "DELAY FOR 150ms"
            n270 = Wait Until Next ms Multiple(millisecond multiple=150) -> ()  [unwired: 1 out]
          }
          frame #28 {
            n271 = call <vilib>:"Bytes At Serial Port.vi"("port number"=w368) -> ("byte count"=w367:u32)  [unwired: 1 out]
            n272 = call <vilib>:"Serial Port Read.vi"("requested byte count"=w367, "port number"=w368) -> ("string read"=w366:string)  [unwired: 1 out]
            n273 = call "GetResponseData.vi"("string read"=w366) -> ("replaced substring"=→"THICKNESS 2":string)  [unwired: 10 in]
          }
          frame #29 {
            n274 = String Length(string="CH1 FREQUENCY CMD") -> (length=w375:i32)
            n275 = Add(x=w375, y=34) -> (x+y=w372:i32)
            n276 = To Byte Integer(number=w372) -> (8bit integer=w373:i8)
            n277 = Type Cast(x=w373) -> (*(type *) &x=w371:string)  [unwired: 1 in]
            n278 = Concatenate Strings(w371, "CH1 FREQUENCY CMD") -> (w369:string)
            "TEMPSTRG 7" <- w369
          }
          frame #30 {
            n279 = String Length(string=w376) -> (length=w377:i32)
            n280 = for {
              N: w377 -> [_]
              tunnel: w376 -> [w381]
              i -> [w384]
              # "BUILD CRC"
              n281 = String To Byte Array(string=w381) -> (unsigned byte array=w380:u8[])
              n282 = for {
                N: 8 -> [_]
                n283 = stacked-sequence {
                  seq-local: [w385 _ _] -> [_ w390 _]
                  frame #0 {
                    # "SAVE CRC"
                    n284 = local read "CRC 11"() -> (w385:i16)
                    n285 = local write "TEMPCRC 5"(w385) -> ()
                  }
                  frame #1 {
                    n286 = Quotient & Remainder(x=w390, y=2) -> (x-y*floor(x/y)=→"x-y*floor(x/y) 5":i32, floor(x/y)=w386:i32)
                    "floor(x/y) 5" <- w386
                    n287 = To Word Integer(number=w386) -> (16bit integer=w388:i16)
                    n288 = local write "CRC 11"(w388) -> ()
                  }
                  frame #2 {
                    w392 = 1
                    n289 = And(x="TEMPCRC 5", y=w392) -> (x .and. y?=w393:i32)
                    n290 = Equal?(x=w393, y=w392) -> (x = y?=w391:bool)
                    n291 = case shown="True" w391 {
                      frame False {
                      }
                      frame True {
                        n292 = local read "CRC 11"() -> (w396:i16)
                        n293 = Exclusive Or(1:8193, 2:w396) -> (0:w395:i32)
                        n294 = To Word Integer(number=w395) -> (16bit integer=w398:i16)
                        n295 = local write "CRC 11"(w398) -> ()
                      }
                    }
                  }
                }
              }
              n296 = Equal To 0?(x=w384) -> (x = 0?=w383:bool)
              n297 = Index Array(array=w380, index=w384) -> (element=w378:u8)
              n298 = case shown="False" w383 {
                tunnel: 16383 -> [_ w404]
                tunnel: w378 -> [w401 w403]
                frame False {
                  n299 = local read "CRC 11"() -> (w400:i16)
                  n300 = Exclusive Or(1:w400, 2:w401) -> (0:w399:i16)
                  n301 = local write "CRC 11"(w399) -> ()
                }
                frame True {
                  n302 = Exclusive Or(1:w404, 2:w403) -> (0:w402:i32)
                  n303 = local write "CRC 11"(w402) -> ()
                }
              }
            }
          }
          frame #31 {
            n304 = And(x="CRC 11", y=16383) -> (x .and. y?=w408:i32)
            n305 = To Word Integer(number=w408) -> (16bit integer=w407:i16)
            n306 = local write "CRC 11"(w407) -> ()
            n307 = Number To Boolean Array(number=w407) -> (Boolean array=w411:bool[])
            "Boolean array 5" <- w411
            n308 = Split 1D Array(array=w411, index=8) -> (first subarray=w406:bool[])  [unwired: 1 out]
          }
          frame #32 {
            n309 = stacked-sequence {
              seq-local: [_ w422 _ _] -> [_ _ w429 _]
              tunnel: w412 -> [w413 _ _ _]
              frame #0 {
                # "FINISH CRC1"
                n310 = Boolean Array To Number(Boolean array=w413) -> (number=w414:u32)
                n311 = And(x=w414, y=127) -> (x .and. y?=w415:u32)
                n312 = To Byte Integer(number=w415) -> (8bit integer=w417:i8)
                n313 = Add(x=w417, y=34) -> (x+y=w419:i32)
                n314 = To Byte Integer(number=w419) -> (8bit integer=w418:i8)
                n315 = Type Cast(x=w418) -> (*(type *) &x=→"CRC1 5":string)  [unwired: 1 in]
              }
              frame #1 {
                # "WORK ON CRC2"
                n316 = local read "CRC 11"() -> (w428:i16)
                n317 = Quotient & Remainder(x=w428, y=128) -> (floor(x/y)=w425:i32)  [unwired: 1 out]
                n318 = To Word Integer(number=w425) -> (16bit integer=w424:i16)
                n319 = Number To Boolean Array(number=w424) -> (Boolean array=w423:bool[])
                n320 = Split 1D Array(array=w423, index=8) -> (first subarray=w422:bool[])  [unwired: 1 out]
              }
              frame #2 {
                # "FINISH CRC2"
                n321 = Boolean Array To Number(Boolean array=w429) -> (number=w430:u32)
                n322 = And(x=w430, y=127) -> (x .and. y?=w437:u32)
                n323 = To Byte Integer(number=w437) -> (8bit integer=w435:i8)
                n324 = Add(x=w435, y=34) -> (x+y=w433:i32)
                n325 = To Byte Integer(number=w433) -> (8bit integer=w434:i8)
                n326 = Type Cast(x=w434) -> (*(type *) &x=→"CRC2 5":string)  [unwired: 1 in]
              }
              frame #3 {
                # "BUILD FINAL MESSAGE HERE"
                n327 = local read "TEMPSTRG 7"() -> (w441:string)
                n328 = local read "CRC1 5"() -> (w440:string)
                n329 = local read "CRC2 5"() -> (w439:string)
                n330 = Concatenate Strings("!", w441, w440, w439) -> (→"COMPLETE MESSAGE 6":string)
              }
            }
          }
          frame #33 {
            n331 = local read "COMPLETE MESSAGE 6"() -> (w444:string)
            n332 = call <vilib>:"Serial Port Write.vi"("string to write"=w444, "port number"=w443) -> ()  [unwired: 1 out]
          }
          frame #34 {
            # "DELAY FOR 150ms"
            n333 = Wait Until Next ms Multiple(millisecond multiple=150) -> ()  [unwired: 1 out]
          }
          frame #35 {
            n334 = call <vilib>:"Bytes At Serial Port.vi"("port number"=w448) -> ("byte count"=w449:u32)  [unwired: 1 out]
            n335 = call <vilib>:"Serial Port Read.vi"("requested byte count"=w449, "port number"=w448) -> ("string read"=w446:string)  [unwired: 1 out]
            n336 = call "GetResponseData.vi"("string read"=w446) -> ("replaced substring"=→"FREQUENCY 1":string)  [unwired: 10 in]
          }
          frame #36 {
            n337 = String Length(string="CH2 FREQUENCY CMD") -> (length=w456:i32)
            n338 = Add(x=w456, y=34) -> (x+y=w453:i32)
            n339 = To Byte Integer(number=w453) -> (8bit integer=w454:i8)
            n340 = Type Cast(x=w454) -> (*(type *) &x=w452:string)  [unwired: 1 in]
            n341 = Concatenate Strings(w452, "CH2 FREQUENCY CMD") -> (w450:string)
            "TEMPSTRG 9" <- w450
          }
          frame #37 {
            n342 = String Length(string=w457) -> (length=w458:i32)
            n343 = for {
              N: w458 -> [_]
              tunnel: w457 -> [w462]
              i -> [w465]
              # "BUILD CRC"
              n344 = String To Byte Array(string=w462) -> (unsigned byte array=w461:u8[])
              n345 = for {
                N: 8 -> [_]
                n346 = stacked-sequence {
                  seq-local: [w466 _ _] -> [_ w471 _]
                  frame #0 {
                    # "SAVE CRC"
                    n347 = local read "CRC 14"() -> (w466:i16)
                    n348 = local write "TEMPCRC 6"(w466) -> ()
                  }
                  frame #1 {
                    n349 = Quotient & Remainder(x=w471, y=2) -> (x-y*floor(x/y)=→"x-y*floor(x/y) 6":i32, floor(x/y)=w467:i32)
                    "floor(x/y) 6" <- w467
                    n350 = To Word Integer(number=w467) -> (16bit integer=w469:i16)
                    n351 = local write "CRC 14"(w469) -> ()
                  }
                  frame #2 {
                    w473 = 1
                    n352 = And(x="TEMPCRC 6", y=w473) -> (x .and. y?=w474:i32)
                    n353 = Equal?(x=w474, y=w473) -> (x = y?=w472:bool)
                    n354 = case shown="True" w472 {
                      frame False {
                      }
                      frame True {
                        n355 = local read "CRC 14"() -> (w477:i16)
                        n356 = Exclusive Or(1:8193, 2:w477) -> (0:w476:i32)
                        n357 = To Word Integer(number=w476) -> (16bit integer=w479:i16)
                        n358 = local write "CRC 14"(w479) -> ()
                      }
                    }
                  }
                }
              }
              n359 = Equal To 0?(x=w465) -> (x = 0?=w464:bool)
              n360 = Index Array(array=w461, index=w465) -> (element=w459:u8)
              n361 = case shown="False" w464 {
                tunnel: 16383 -> [_ w485]
                tunnel: w459 -> [w482 w484]
                frame False {
                  n362 = local read "CRC 14"() -> (w481:i16)
                  n363 = Exclusive Or(1:w481, 2:w482) -> (0:w480:i16)
                  n364 = local write "CRC 14"(w480) -> ()
                }
                frame True {
                  n365 = Exclusive Or(1:w485, 2:w484) -> (0:w483:i32)
                  n366 = local write "CRC 14"(w483) -> ()
                }
              }
            }
          }
          frame #38 {
            n367 = And(x="CRC 14", y=16383) -> (x .and. y?=w489:i32)
            n368 = To Word Integer(number=w489) -> (16bit integer=w486:i16)
            n369 = Number To Boolean Array(number=w486) -> (Boolean array=w492:bool[])
            "Boolean array 6" <- w492
            n370 = Split 1D Array(array=w492, index=8) -> (first subarray=w488:bool[])  [unwired: 1 out]
          }
          frame #39 {
            n371 = stacked-sequence {
              seq-local: [_ w503 _ _] -> [_ _ w510 _]
              tunnel: w493 -> [w494 _ _ _]
              frame #0 {
                # "FINISH CRC1"
                n372 = Boolean Array To Number(Boolean array=w494) -> (number=w495:u32)
                n373 = And(x=w495, y=127) -> (x .and. y?=w496:u32)
                n374 = To Byte Integer(number=w496) -> (8bit integer=w498:i8)
                n375 = Add(x=w498, y=34) -> (x+y=w500:i32)
                n376 = To Byte Integer(number=w500) -> (8bit integer=w499:i8)
                n377 = Type Cast(x=w499) -> (*(type *) &x=→"CRC1 6":string)  [unwired: 1 in]
              }
              frame #1 {
                # "WORK ON CRC2"
                n378 = local read "CRC 14"() -> (w509:i16)
                n379 = Quotient & Remainder(x=w509, y=128) -> (floor(x/y)=w506:i32)  [unwired: 1 out]
                n380 = To Word Integer(number=w506) -> (16bit integer=w505:i16)
                n381 = Number To Boolean Array(number=w505) -> (Boolean array=w504:bool[])
                n382 = Split 1D Array(array=w504, index=8) -> (first subarray=w503:bool[])  [unwired: 1 out]
              }
              frame #2 {
                # "FINISH CRC2"
                n383 = Boolean Array To Number(Boolean array=w510) -> (number=w511:u32)
                n384 = And(x=w511, y=127) -> (x .and. y?=w518:u32)
                n385 = To Byte Integer(number=w518) -> (8bit integer=w516:i8)
                n386 = Add(x=w516, y=34) -> (x+y=w514:i32)
                n387 = To Byte Integer(number=w514) -> (8bit integer=w515:i8)
                n388 = Type Cast(x=w515) -> (*(type *) &x=→"CRC2 6":string)  [unwired: 1 in]
              }
              frame #3 {
                # "BUILD FINAL MESSAGE HERE"
                n389 = local read "TEMPSTRG 9"() -> (w522:string)
                n390 = local read "CRC1 6"() -> (w521:string)
                n391 = local read "CRC2 6"() -> (w520:string)
                n392 = Concatenate Strings("!", w522, w521, w520) -> (→"COMPLETE MESSAGE 9":string)
              }
            }
          }
          frame #40 {
            n393 = local read "COMPLETE MESSAGE 9"() -> (w525:string)
            n394 = call <vilib>:"Serial Port Write.vi"("string to write"=w525, "port number"=w524) -> ()  [unwired: 1 out]
          }
          frame #41 {
            # "DELAY FOR 150ms"
            n395 = Wait Until Next ms Multiple(millisecond multiple=150) -> ()  [unwired: 1 out]
          }
          frame #42 {
            n396 = call <vilib>:"Bytes At Serial Port.vi"("port number"=w529) -> ("byte count"=w530:u32)  [unwired: 1 out]
            n397 = call <vilib>:"Serial Port Read.vi"("requested byte count"=w530, "port number"=w529) -> ("string read"=w528:string)  [unwired: 1 out]
            n398 = call "GetResponseData.vi"("string read"=w528) -> ("replaced substring"=→"FREQUENCY 2":string)  [unwired: 10 in]
          }
          frame #43 {
            # "Shutter Status"
            n399 = stacked-sequence {
              tunnel: w531 -> [w533 _ w539]
              frame #0 {
                # "Request Shutter Status"
                n400 = call <vilib>:"Serial Port Write.vi"("string to write"="!$U?[T", "port number"=w533) -> ()  [unwired: 1 out]
              }
              frame #1 {
                n401 = Wait Until Next ms Multiple(millisecond multiple=150) -> ()  [unwired: 1 out]
              }
              frame #2 {
                # "Get & Display Shutter Status"
                n402 = call <vilib>:"Bytes At Serial Port.vi"("port number"=w539) -> ("byte count"=w540:u32)  [unwired: 1 out]
                n403 = call <vilib>:"Serial Port Read.vi"("requested byte count"=w540, "port number"=w539) -> ("string read"=w542:string)  [unwired: 1 out]
                n404 = String Subset(string=w542, offset (0)=3, length (rest)=1 ("length (rest)")) -> (substring=w537:string)
                n405 = Hexadecimal String To Number(string=w537) -> (number=w536:u32)  [unwired: 2 in, 1 out]
                n406 = Not Equal To 0?(x=w536) -> (x != 0?=→"Shutter":bool)
              }
            }
          }
        }
      }
    }
  }
